vi "E-Stop Test.vi"(8 "error in":errorcluster, 10 "State":T1, 11 "Light Stack in":refnum<class "Light Stack.lvclass">) -> (0 "error out":errorcluster, 2 "Output State":T1, 3 "Light Stack out":refnum<class "Light Stack.lvclass">)   [LabVIEW 2018, in "Light Stack.lvlib" / "Light Stack.lvclass"]
uses:
  Light Stack.lvclass
  Custom Controls/Light Mode.ctl
  Custom Controls/Light Select.ctl
  Light Stack.lvclass/Light Stack.ctl
  Light Stack.lvlib
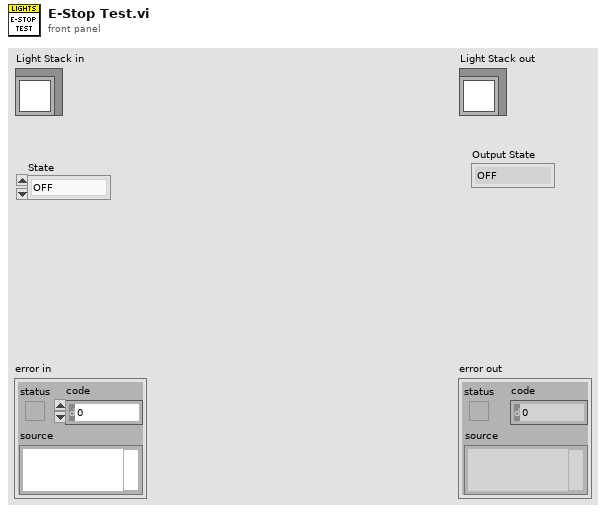
[diagram p1: front panel]
types:
  T1 = typedef "Light Stack.lvlib/Light Mode.ctl" = enum16{"OFF", "ON", "BLINK"}
  T2 = typedef "Light Stack.lvlib/Light Select.ctl" = enum16{"Red", "Amber", "Green", "Blue"}
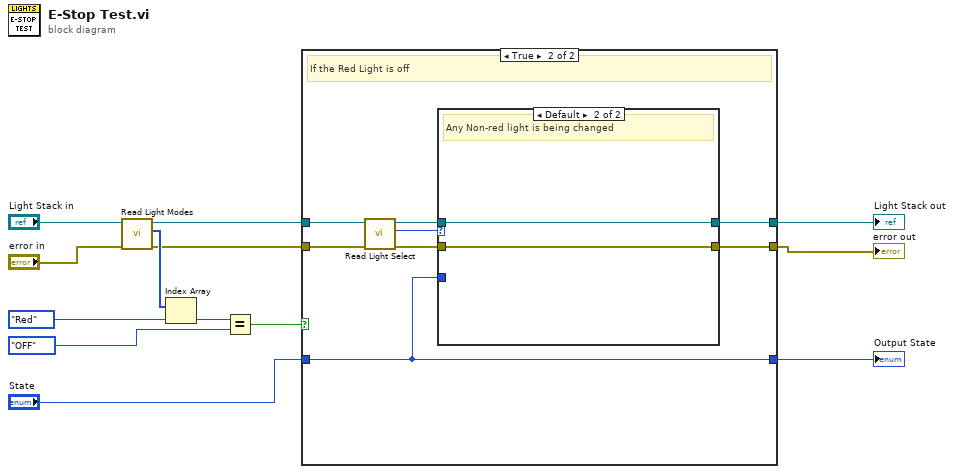
[diagram p0: block diagram]
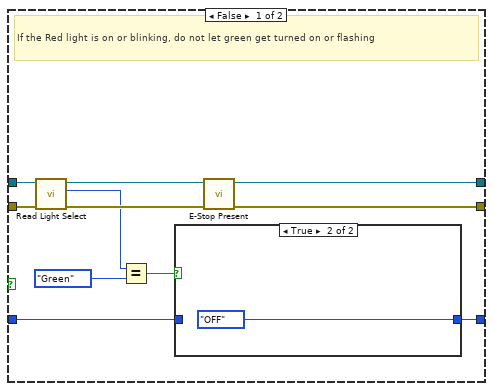
[diagram p2: hidden frame]
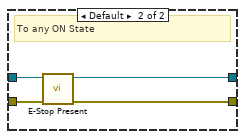
[diagram p5: hidden frame]
diagram:
  n1 = call "Read Light Modes.vi"("error in (no error)"="error in", "Light Stack in"="Light Stack in") -> ("error out"=w5:errorcluster, "Light Modes"=w6:T1[], "Light Stack out"=w3:refnum<class "Light Stack.lvclass">)  [unwired: 7 in]
  n2 = Index Array(array=w6, index=Light_Select."Red" ("State")) -> (element=w13:T1)
  n3 = Equal?(x=w13, y=Light_Mode."OFF" ("Light Select")) -> (x = y?=w12:bool)
  n4 = case shown="True" w12 {
    tunnel: "State" -> [w20 w27]
    tunnel: [w19 w27] -> w10
    tunnel: w3 -> [w23 w34]
    tunnel: w5 -> [w24 w33]
    tunnel: [w17 w29] -> w9
    tunnel: [w15 w28] -> w8
    frame False {
      # "If the Red light is on or blinking, do not let green get turned on or flashing"
      n5 = call "Read Light Select.vi"("error in (no error)"=w24, "Light Stack in"=w23) -> ("error out"=w16:errorcluster, "Light Select"=w14:T2, "Light Stack out"=w18:refnum<class "Light Stack.lvclass">)  [unwired: 7 in]
      n6 = Equal?(x=w14, y=Light_Select."Green" ("Light Select")) -> (x = y?=w21:bool)
      n7 = case shown="True" w21 {
        tunnel: w20 -> [w25 _]
        tunnel: [w25 Light_Mode."OFF" ("State")] -> w19
        frame False {
        }
        frame True {
        }
      }
      n8 = call "E-Stop Present.vi"("error in"=w16, "Light Stack in"=w18) -> ("error out"=w15:errorcluster, "Light Stack out"=w17:refnum<class "Light Stack.lvclass">)  [unwired: 8 in]
    }
    frame True {
      # "If the Red Light is off"
      n9 = call "Read Light Select.vi"("error in (no error)"=w33, "Light Stack in"=w34) -> ("error out"=w30:errorcluster, "Light Select"=w32:T2, "Light Stack out"=w31:refnum<class "Light Stack.lvclass">)  [unwired: 7 in]
      n10 = case shown="Default" w32 {
        tunnel: w31 -> [w39 w47]
        tunnel: w30 -> [w36 w46]
        tunnel: [w37 w47] -> w29
        tunnel: [w35 w46] -> w28
        tunnel: w27 -> [w38 _]
        frame "Red" {
          # "If the red light is getting changed:"
          n11 = case shown="\"OFF\"" w38 {
            tunnel: w39 -> [w41 w44]
            tunnel: [w41 w43] -> w37
            tunnel: w36 -> [w40 w45]
            tunnel: [w40 w42] -> w35
            frame "OFF" {
              # "To Off, No Estop Necessary"
            }
            frame Default {
              # "To any ON State"
              n12 = call "E-Stop Present.vi"("error in"=w45, "Light Stack in"=w44) -> ("error out"=w42:errorcluster, "Light Stack out"=w43:refnum<class "Light Stack.lvclass">)  [unwired: 8 in]
            }
          }
        }
        frame Default {
          # "Any Non-red light is being changed"
        }
      }
    }
  }
  "error out" <- w8
  "Light Stack out" <- w9
  "Output State" <- w10
